vi "Retention Test Multiple.vi"(5 "Current address":i32, 6 "WL voltage (V)":dbl, 7 "target outfile":path, 8 "error in (no error)":errorcluster, 9 "final resistance (ohm)":dbl, 10 "SL voltage (V)":dbl, 11 "IVI Refnum in":refnum<k15>) -> (0 "error out":errorcluster, 3 "IVI Refnum out":refnum<k15>)   [LabVIEW 2018]
uses:
  <vilib>/Utility/file.llb/Write Delimited Spreadsheet (DBL).vi
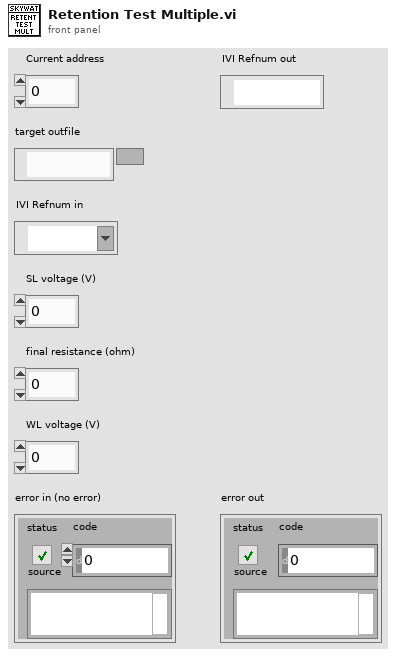
[diagram p1: front panel]
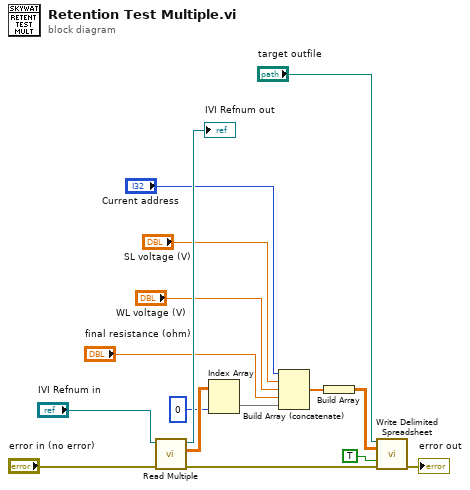
[diagram p0: block diagram]
diagram:
  n1 = call "Read Multiple.vi"("error in (no error)"="error in (no error)", "instrument handle"="IVI Refnum in") -> ("error out"=w8:errorcluster, "resistances (ohm)"=w3:dbl[][], "instrument handle out"=→"IVI Refnum out":refnum<k15>)  [unwired: 6 in, 1 out]
  n2 = Index Array(array=w3, index (col)=0 ("disabled index (col)")) -> (element=w2:dbl[])  [unwired: 1 in]
  n3 = Build Array (concatenate)("Current address", "SL voltage (V)", "WL voltage (V)", "final resistance (ohm)", w2) -> (w4:dbl[])
  n4 = Build Array(w4) -> (w5:dbl[][])
  n5 = call-poly <vilib>:"Write Delimited Spreadsheet.vi"("file path (dialog if empty)"="target outfile", "2D data"=w5, "append to file? (new file:F)"=TRUE, "error in (no error)"=w8) -> ("error out"=→"error out":errorcluster)  [unwired: 10 in, 1 out]
